vi "7.1-Functional Global for Forbrain Act Data.vi"(1 "6.1.11-Forebrain Act Neuron Data":T1, 2 "Command":T3(ring)) -> (0 "6.1.11-Outputted Forebrain Act Neuron Data":T1)   [LabVIEW 2010]
uses:
  6-OCU Neurons/6.1.11- Forbrain and midbrain Act neuron.ctl
  4-High Neurons/4.1-Midbrain Act Data.ctl
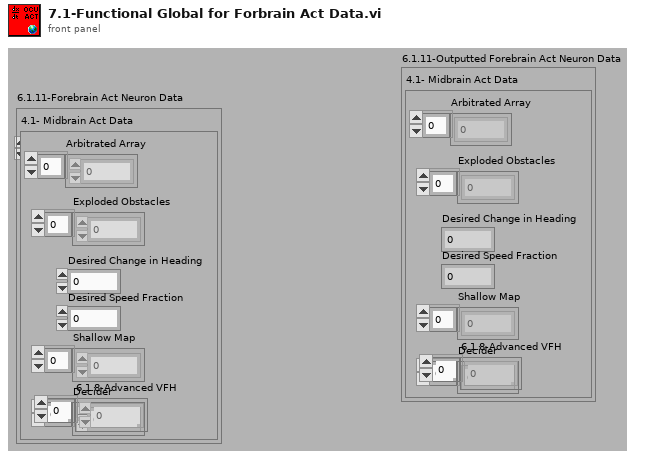
[diagram p1: front panel]
types:
  T1 = typedef "6.1.11- Forbrain and midbrain Act neuron.ctl" = cluster{"4.1- Midbrain Act Data":T2, "6.1.8-Advanced VFH":dbl[]}
  T2 = typedef "4.1-Midbrain Act Data.ctl" = cluster{"Arbitrated Array":sgl[], "Exploded Obstacles":sgl[], "Desired Change in Heading":sgl, "Desired Speed Fraction":sgl, "Shallow Map":dbl[], "Decider":dbl[]}
  T3 = enum16{"Set Forbrain Act Data", "Read Forebrain Act Data"}
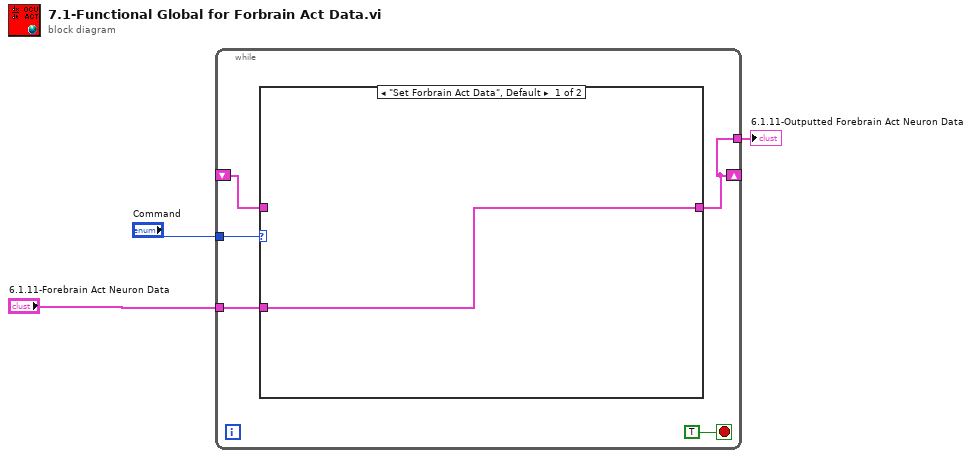
[diagram p0: block diagram]
diagram:
  n1 = while {
    shift-right: [w4] -> _
    shift-left: _ -> [w5]
    tunnel: "Command" -> [w7]
    tunnel: "6.1.11-Forebrain Act Neuron Data" -> [w6]
    tunnel: [w4] -> w1
    stop <- TRUE stop-if-true
    n2 = case shown="\"Set Forbrain Act Data\", Default" w7 {
      tunnel: [w9 w10] -> w4
      tunnel: w6 -> [w9 _]
      tunnel: w5 -> [_ w10]
      frame "Set Forbrain Act Data", Default {
      }
      frame "Read Forebrain Act Data" {
      }
    }
  }
  "6.1.11-Outputted Forebrain Act Neuron Data" <- w1
